vi "PYTHON UTIL Format Error Code__ogtk.vi"(3 "lineno":i32, 4 "error in (no error)":errorcluster, 5 "message":string, 6 "code":i32, 7 "Bool32":i32) -> (0 "error out":errorcluster)   [LabVIEW 2010]
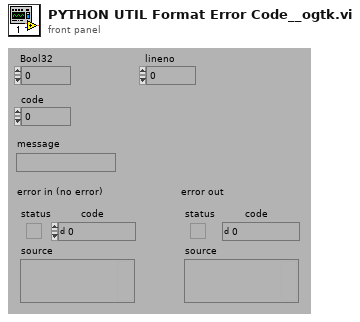
[diagram p1: front panel]
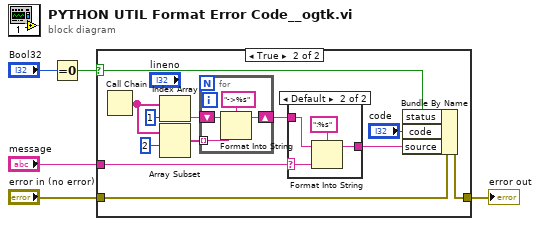
[diagram p0: block diagram]
diagram:
  n1 = Equal To 0?(x="Bool32") -> (x = 0?=w5:bool)
  n2 = case shown="True" w5 {
    selector: w5 -> [_ w16]
    tunnel: "error in (no error)" -> [w6 w18]
    tunnel: [w6 w17] -> w4
    tunnel: "message" -> [_ w8]
    frame False {
    }
    frame True {
      n3 = Call Chain() -> (call chain=w13:string[])
      n4 = Index Array(array=w13, index=1 ("Index")) -> (element=w11:string)
      n5 = Array Subset(array=w13, index=2 ("Length")) -> (w10:string[])  [unwired: 1 in]
      n6 = for {
        shift-right: [w25] -> w9
        shift-left: w11 -> [w27]
        tunnel: w10 -> [w26] mode=indexing
        n7 = Format Into String(format string="->%s" ("Format String"), initial string=w27, w26) -> (resulting string=w25:string)  [unwired: 1 in, 1 out]
      }
      n8 = case shown="Default" w8 {
        selector: w8 -> [_ w21]
        tunnel: w9 -> [w19 w23]
        tunnel: [w19 w22] -> w7
        frame "" {
        }
        frame Default {
          n9 = Format Into String(format string=":%s" ("Format String"), initial string=w23, w21) -> (resulting string=w22:string)  [unwired: 1 in, 1 out]
        }
      }
      n10 = Bundle By Name(cluster=w18, "status"=w16, "code"="code", "source"=w7) -> (w17:errorcluster)
    }
  }
  "error out" <- w4
